vi "AI_client.vi"() -> ()   [LabVIEW 2017]
panel:
  out "times":i32
  out "timeout times":dbl
  out "timeflow":u32[](graph)
  in  "image path":path
  out "Average Runtime":dbl
  in  "test_times":dbl=20.0
  out "PASS":dbl
  out "Complete":bool
  out "pwd vert":bool
  out "AIT":bool
  in  "error in":errorcluster
  out "error out":errorcluster
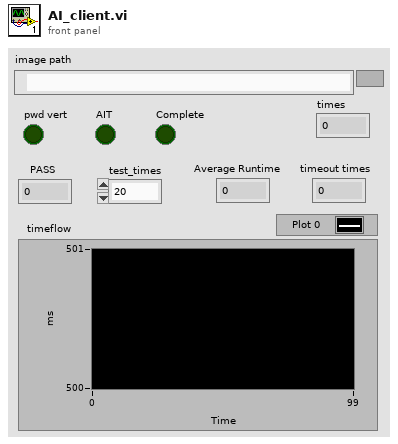
[diagram p1: front panel]
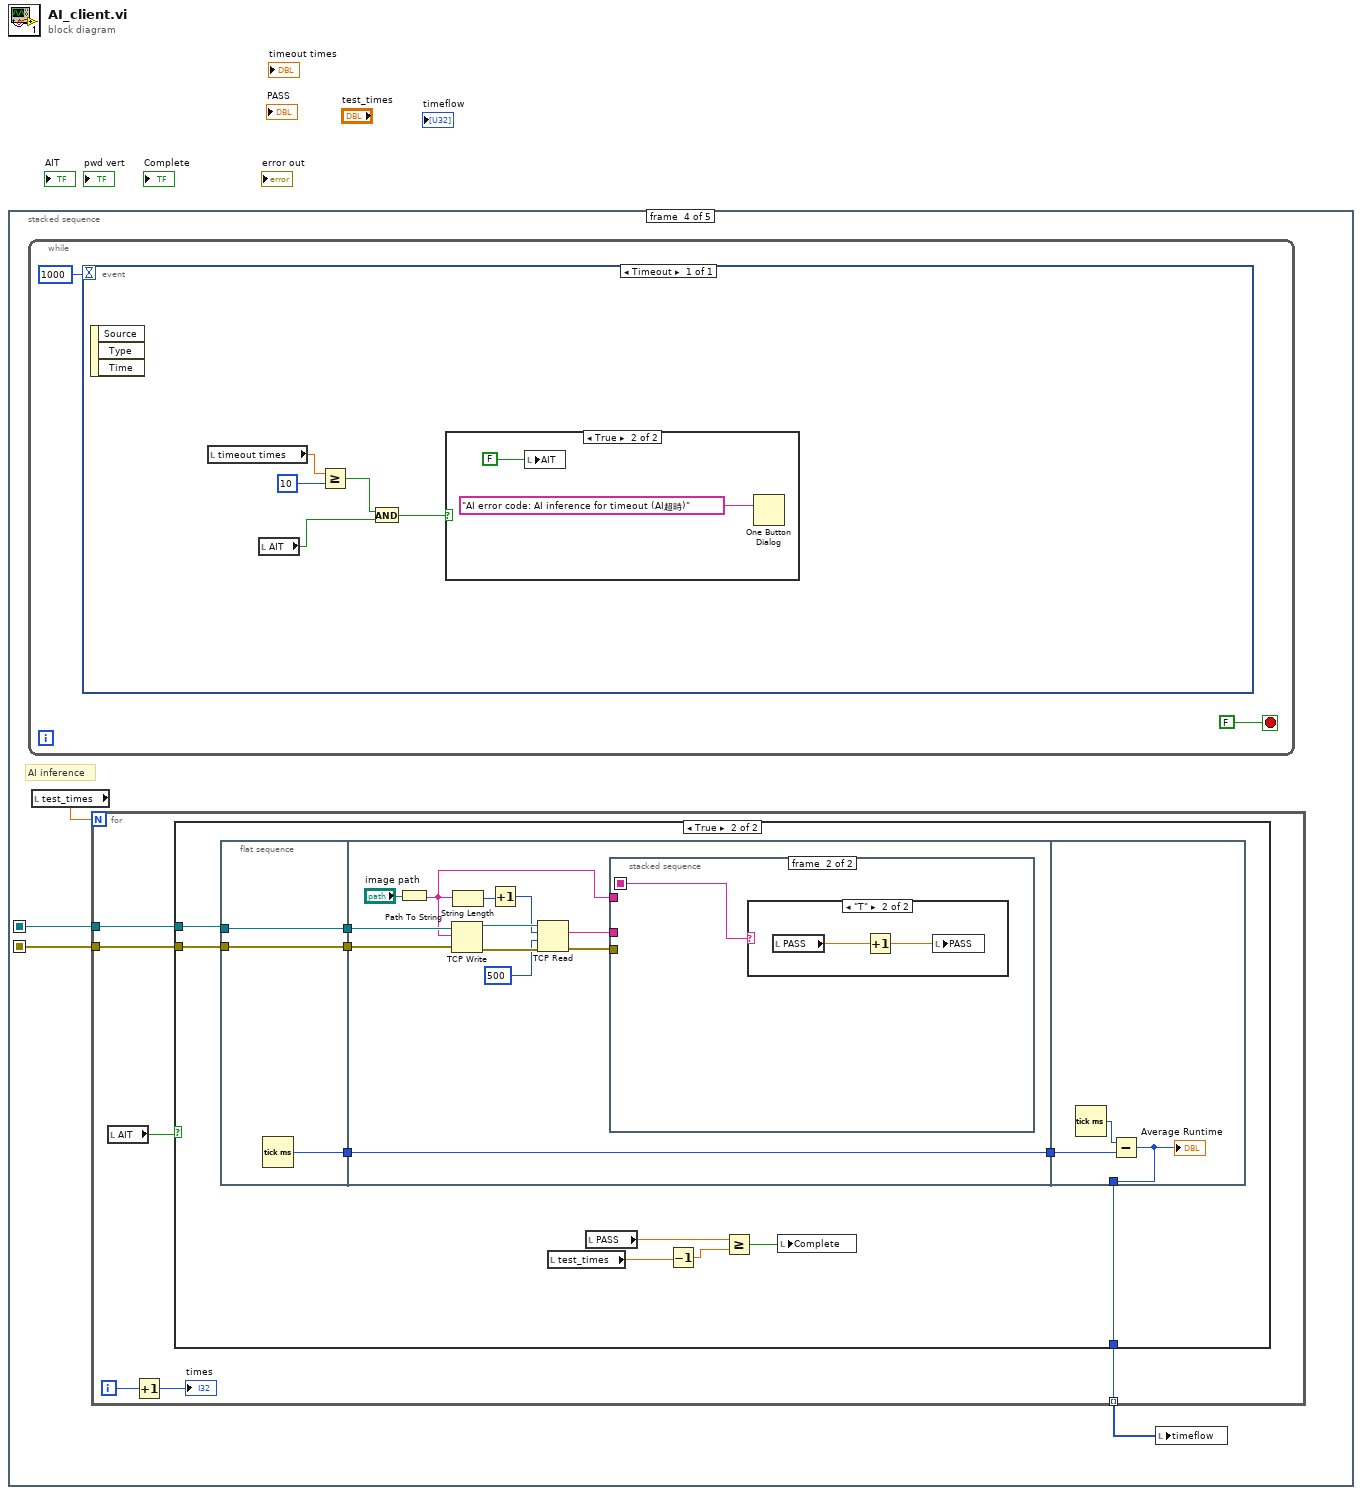
[diagram p0: block diagram]
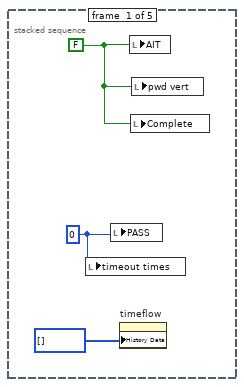
[diagram p2: hidden frame]
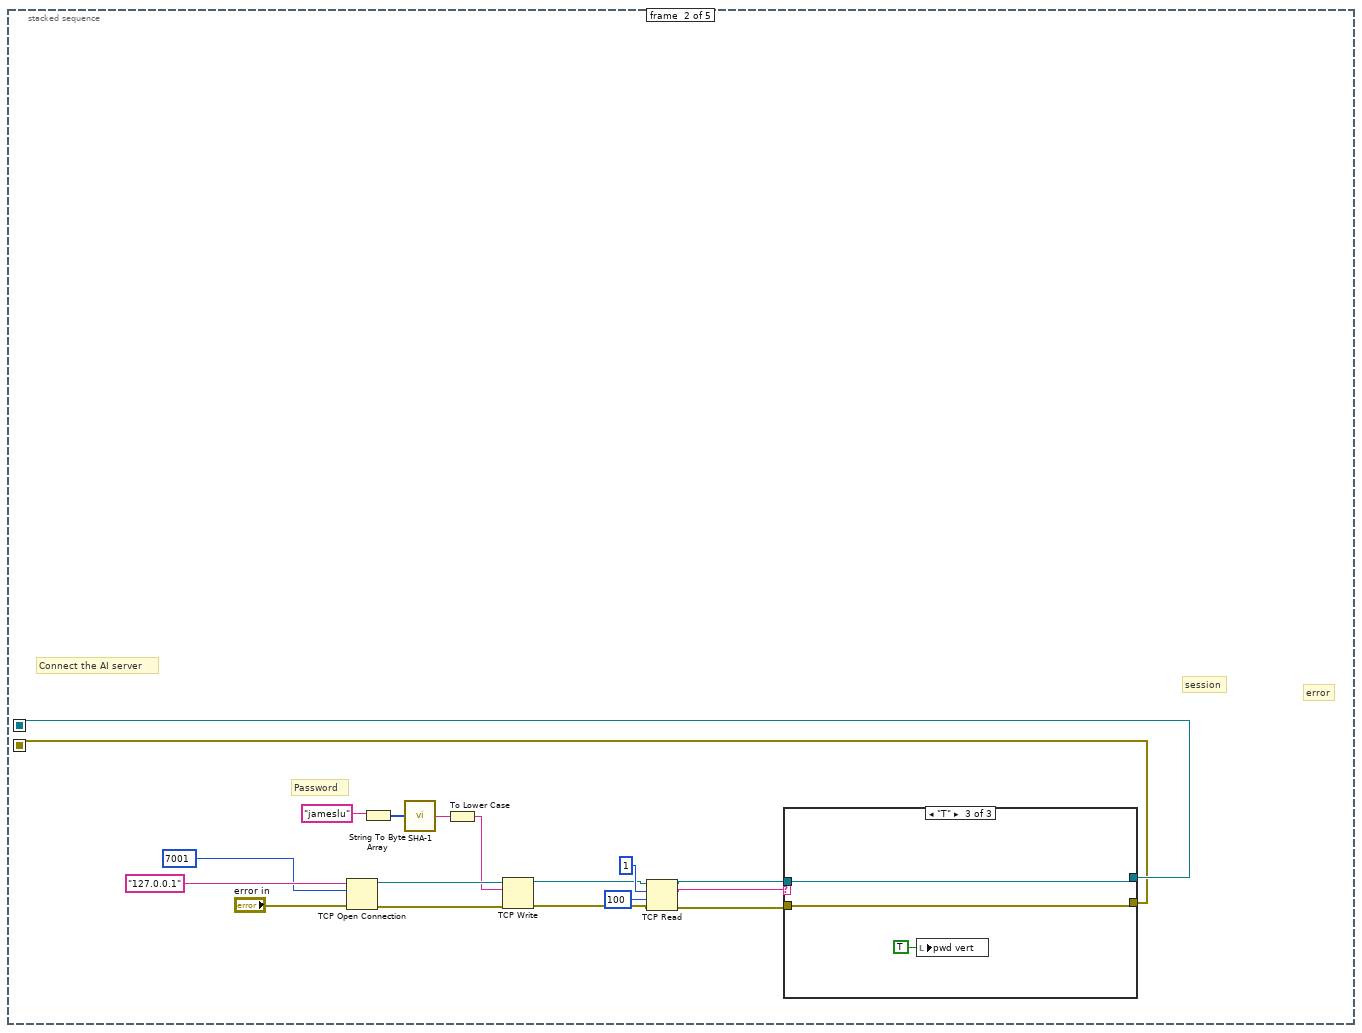
[diagram p3: hidden frame]
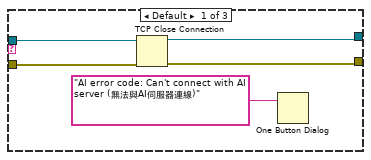
[diagram p4: hidden frame]
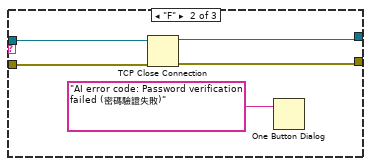
[diagram p5: hidden frame]
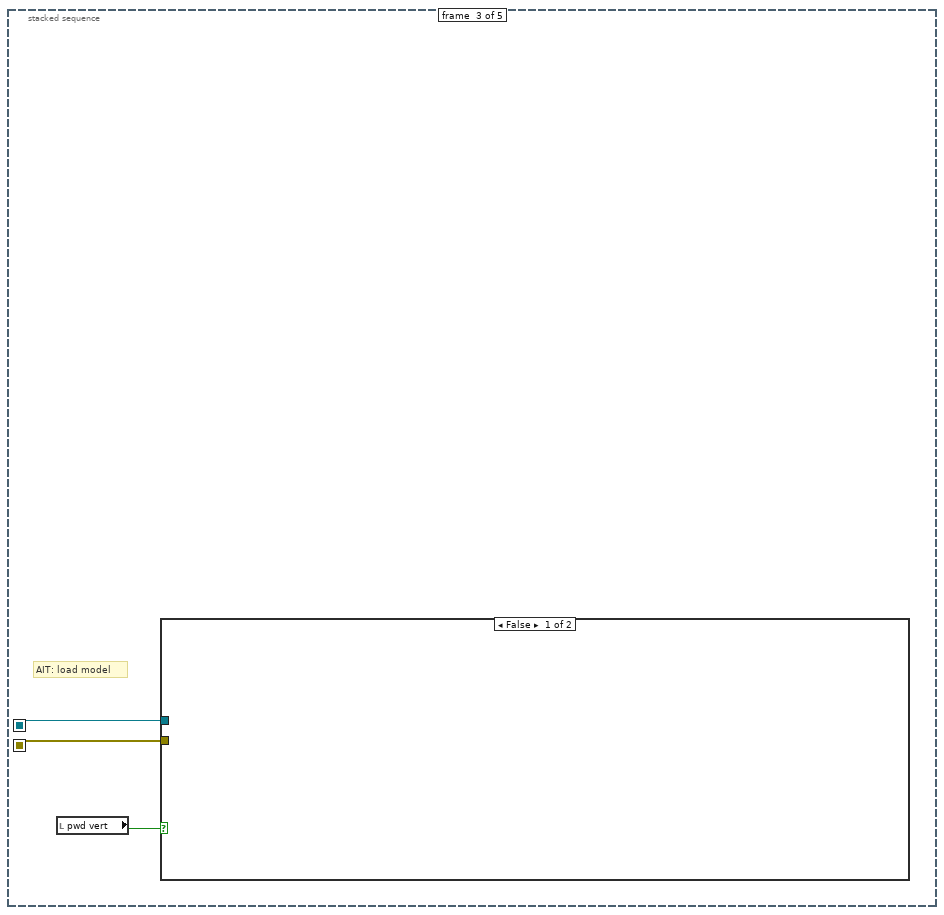
[diagram p6: hidden frame]
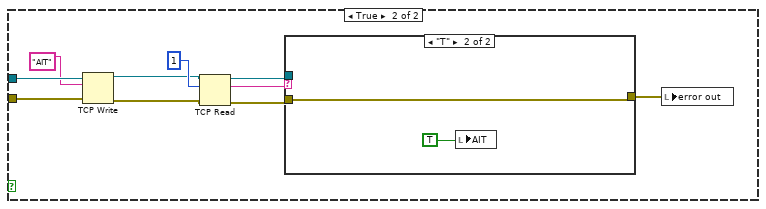
[diagram p7: hidden frame]
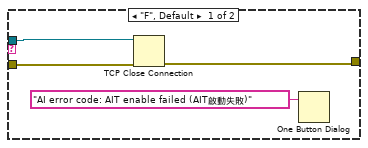
[diagram p8: hidden frame]
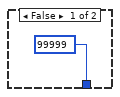
[diagram p9: hidden frame]
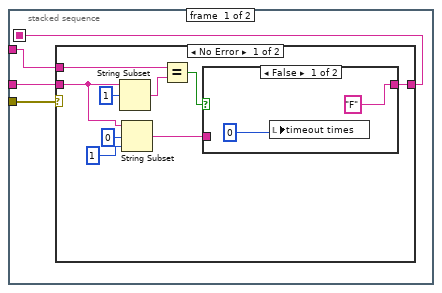
[diagram p10: hidden frame]
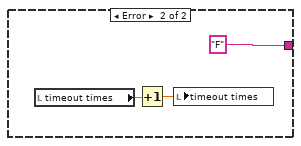
[diagram p12: hidden frame]
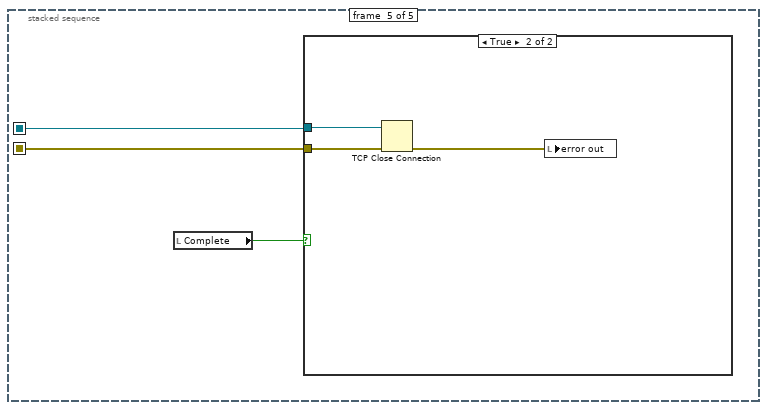
[diagram p15: hidden frame]
diagram:
  n1 = stacked-sequence {
    seq-local: [_ w11 _ _ _] -> [_ _ w36 w56 w127]
    seq-local: [_ w12 _ _ _] -> [_ _ w37 w57 w125]
    frame #0 {
      w1 = 0
      w3 = FALSE
      n2 = local write "timeout times"(w1) -> ()
      n3 = local write "PASS"(w1) -> ()
      n4 = property on="timeflow" class="WFChart (strict)"("History Data"=u32[] []) -> ()  [unwired: 2 in, 2 out]
      n5 = local write "AIT"(w3) -> ()
      n6 = local write "Complete"(w3) -> ()
      n7 = local write "pwd vert"(w3) -> ()
    }
    frame #1 {
      # "Connect the AI server"
      # "session"
      # "error"
      # "Password"
      n8 = TCP Open Connection(address="127.0.0.1", remote port or service name=7001, error in (no error)="error in") -> (connection ID=w17:refnum<k5>, error out=w16:errorcluster)  [unwired: 2 in]
      n9 = String To Byte Array(string="jameslu" ("data in")) -> (unsigned byte array=w20:u8[])
      n10 = call "SHA-1.vi"("Data"=w20) -> ("output"=w14:string)
      n11 = To Lower Case(string=w14) -> (all lower case string=w13:string)
      n12 = TCP Write(connection ID=w17, data in=w13, error in (no error)=w16) -> (connection ID out=w8:refnum<k5>, error out=w7:errorcluster)  [unwired: 1 in, 1 out]
      n13 = TCP Read(connection ID=w8, bytes to read=1, error in (no error)=w7, 9:100 ("timeout ms (25000)")) -> (connection ID out=w4:refnum<k5>, data out=w5:string, error out=w6:errorcluster)  [unwired: 1 in]
      n14 = case shown="\"T\"" w5 {
        tunnel: w4 -> [w26 w31 w33]
        tunnel: [w24 w28 w33] -> w12
        tunnel: w6 -> [w25 w30 w32]
        tunnel: [w23 w29 w32] -> w11
        frame Default {
          n15 = TCP Close Connection(connection ID=w26, error in (no error)=w25) -> (connection ID out=w24:refnum<k5>, error out=w23:errorcluster)  [unwired: 1 in]
          n16 = One Button Dialog(message="AI error code: Can't connect with AI server (無法與AI伺服器連線)") -> ()  [unwired: 1 in, 1 out]
        }
        frame "F" {
          n17 = TCP Close Connection(connection ID=w31, error in (no error)=w30) -> (connection ID out=w28:refnum<k5>, error out=w29:errorcluster)  [unwired: 1 in]
          n18 = One Button Dialog(message="AI error code: Password verification failed (密碼驗證失敗)") -> ()  [unwired: 1 in, 1 out]
        }
        frame "T" {
          n19 = local write "pwd vert"(TRUE) -> ()
        }
      }
    }
    frame #2 {
      # "AIT: load model"
      n20 = local read "pwd vert"() -> (w35:bool)
      n21 = case shown="False" w35 {
        tunnel: w37 -> [_ w47]
        tunnel: w36 -> [_ w46]
        frame False {
        }
        frame True {
          n22 = TCP Write(connection ID=w47, data in="AIT", error in (no error)=w46) -> (connection ID out=w41:refnum<k5>, error out=w42:errorcluster)  [unwired: 1 in, 1 out]
          n23 = TCP Read(connection ID=w41, bytes to read=1, error in (no error)=w42) -> (connection ID out=w39:refnum<k5>, data out=w38:string, error out=w40:errorcluster)  [unwired: 2 in]
          n24 = case shown="\"T\"" w38 {
            tunnel: w39 -> [w51 _]
            tunnel: w40 -> [w50 w53]
            tunnel: [w48 w53] -> w44
            frame "F", Default {
              n25 = TCP Close Connection(connection ID=w51, error in (no error)=w50) -> (error out=w48:errorcluster)  [unwired: 1 in, 1 out]
              n26 = One Button Dialog(message="AI error code: AIT enable failed (AIT啟動失敗)") -> ()  [unwired: 1 in, 1 out]
            }
            frame "T" {
              n27 = local write "AIT"(TRUE) -> ()
            }
          }
          n28 = local write "error out"(w44) -> ()
        }
      }
    }
    frame #3 {
      # "AI inference"
      n29 = while {
        stop <- FALSE stop-if-true
        n30 = event shown="[0] Timeout" {
          selector: _ -> [_]
          dyn-events: _ -> [_]
          timeout: 1000 -> [_]
          event Timeout {
            n31 = event-data() -> ()  [unwired: 1 in, 3 out]
            n32 = local read "timeout times"() -> (w122:dbl)
            n33 = local read "AIT"() -> (w119:bool)
            n34 = Greater Or Equal?(x=w122, y=10) -> (x >= y?=w120:bool)
            n35 = And(x=w120, y=w119) -> (x .and. y?=w118:bool)
            n36 = case shown="True" w118 {
              frame False {
              }
              frame True {
                n37 = local write "AIT"(FALSE) -> ()
                n38 = One Button Dialog(message="AI error code: AI inference for timeout (AI超時)") -> ()  [unwired: 1 in, 1 out]
              }
            }
          }
        }
      }
      n39 = local read "test_times"() -> (w55:dbl)
      n40 = for {
        N: w55 -> [_]
        tunnel: w57 -> [w63]
        tunnel: w56 -> [w62]
        tunnel: [w60] -> w54 mode=indexing
        i -> [w59]
        n41 = local read "AIT"() -> (w61:bool)
        n42 = Increment(x=w59) -> (x+1=→"times":i32)
        n43 = case shown="True" w61 {
          tunnel: w63 -> [_ w71]
          tunnel: [99999 w66] -> w60
          tunnel: w62 -> [_ w65]
          frame False {
          }
          frame True {
            n44 = flat-sequence {
              tunnel: w71 -> [w78]
              tunnel: [w78] -> w75
              tunnel: [w77] -> w74
              tunnel: w65 -> [w76]
              tunnel: [w76] -> w73
              tunnel: w75 -> [w90]
              tunnel: [w87] -> w72
              tunnel: w74 -> [w87]
              tunnel: w73 -> [w82]
              tunnel: w72 -> [w114]
              tunnel: [w113] -> w66
              frame #0 {
                n45 = Tick Count (ms)() -> (millisecond timer value=w77:u32)
              }
              frame #1 {
                n46 = Path To String(path="image path") -> (string=w79:string)
                n47 = TCP Write(connection ID=w90, data in=w79, error in (no error)=w82) -> (connection ID out=w89:refnum<k5>, error out=w88:errorcluster)  [unwired: 1 in, 1 out]
                n48 = String Length(string=w79) -> (length=w81:i32)
                n49 = Increment(x=w81) -> (x+1=w80:i32)
                n50 = TCP Read(connection ID=w89, bytes to read=w80, error in (no error)=w88, 9:500 ("bytes to read")) -> (data out=w84:string, error out=w83:errorcluster)  [unwired: 1 in, 1 out]
                n51 = stacked-sequence {
                  seq-local: [w92 _] -> [_ w110]
                  tunnel: w83 -> [w94 _]
                  tunnel: w84 -> [w93 _]
                  tunnel: w79 -> [w91 _]
                  frame #0 {
                    n52 = case shown="No Error" w94 {
                      tunnel: w93 -> [w97 _]
                      tunnel: [w95 "F" ("data out")] -> w92
                      tunnel: w91 -> [w103 _]
                      frame No Error {
                        n53 = String Subset(string=w97, offset (0)=1) -> (substring=w100:string)  [unwired: 1 in]
                        n54 = String Subset(string=w97, offset (0)=0, length (rest)=1 ("length (rest)")) -> (substring=w96:string)
                        n55 = Equal?(x=w103, y=w100) -> (x = y?=w101:bool)
                        n56 = case shown="False" w101 {
                          tunnel: w96 -> [_ w106]
                          tunnel: ["F" ("data out") w106] -> w95
                          frame False {
                            n57 = local write "timeout times"(0) -> ()
                          }
                          frame True {
                          }
                        }
                      }
                      frame Error {
                        n58 = local read "timeout times"() -> (w109:dbl)
                        n59 = Increment(x=w109) -> (x+1=w108:dbl)
                        n60 = local write "timeout times"(w108) -> ()
                      }
                    }
                  }
                  frame #1 {
                    n61 = case shown="\"T\"" w110 {
                      frame "F", Default {
                      }
                      frame "T" {
                        n62 = local read "PASS"() -> (w111:dbl)
                        n63 = Increment(x=w111) -> (x+1=w112:dbl)
                        n64 = local write "PASS"(w112) -> ()
                      }
                    }
                  }
                }
              }
              frame #2 {
                n65 = Tick Count (ms)() -> (millisecond timer value=w115:u32)
                n66 = Subtract(x=w115, y=w114) -> (x-y=w113:u32)
                "Average Runtime" <- w113
              }
            }
            n67 = local read "test_times"() -> (w68:dbl)
            n68 = local read "PASS"() -> (w69:dbl)
            n69 = Decrement(x=w68) -> (x-1=w67:dbl)
            n70 = Greater Or Equal?(x=w69, y=w67) -> (x >= y?=w70:bool)
            n71 = local write "Complete"(w70) -> ()
          }
        }
      }
      n72 = local write "timeflow"(w54) -> ()
    }
    frame #4 {
      n73 = local read "Complete"() -> (w126:bool)
      n74 = case shown="True" w126 {
        tunnel: w127 -> [_ w129]
        tunnel: w125 -> [_ w130]
        frame False {
        }
        frame True {
          n75 = TCP Close Connection(connection ID=w130, error in (no error)=w129) -> (error out=w128:errorcluster)  [unwired: 1 in, 1 out]
          n76 = local write "error out"(w128) -> ()
        }
      }
    }
  }
